vi "Photodetector DAQ (temp).vi"() -> ()   [LabVIEW 2018]
uses:
  <vilib>/DAQmx/read.llb/DAQmx Read (Analog 1D Wfm NChan NSamp).vi
  <vilib>/Analysis/8numeric.llb/1D Numeric Integration.vi
  <vilib>/DAQmx/create/channels.llb/DAQmx Create Channel (AI-Voltage-Basic).vi
  <vilib>/DAQmx/configure/timing.llb/DAQmx Timing (Sample Clock).vi
  <vilib>/DAQmx/configure/trigger.llb/DAQmx Start Trigger (Digital Edge).vi
  <vilib>/DAQmx/miscellaneous.llb/DAQmx Fill In Error Info.vi
  <vilib>/Waveform/WDTOps.llb/WDT Index Channel by Name DBL.vi
  <vilib>/Analysis/NI_AALPro.lvlib
panel:
  out "Minimum of absorption signal":dbl[](graph)
  out "Integral of PMT signal":dbl[](graph)
  out "Waveform Graph":waveform(dbl)[](graph)
  in  "Save data?":bool
  in  "file path (dialog if empty)":path=path "C:/Users/Oskari/Google Drive/CeNTREX Oskari/TlF beam profiling/Data acquisition software/LabView/test.csv"
  out "Error message message":string=" INSTRUCTIONS:\r\rNormal Use:  When using subVIs that incorporate the error in/error out (or error I/O) structure, place this handler where you want to inform the user of an error, typically at the end of the I/O data path, as the last action of the program.  If the error in error? is ERROR, the handler creates a message describing the error and its source.  If the type of dialog = 1 (default), the message is displayed to the user, who can only acknowedge it.  If the type = 2, the user can acknowledge the message or abort execution; aborting a program with active I/O is not recommended.  If the type = 0, no message is displayed; this is used to process the error programmatically, and the error out cluster elements are wired to individual terminals for that reason.  \r\rOther Use:\n\r\nlocal testing.  To test the error code of a subVI or function that does not have the error I/O structure, you can wire its error code and a source string to the local error code and error source inputs.  If error in error? indicates no error and error code is not equal to 0, the local code and source are substituted for the error in values, and error? is set TRUE (ERROR)."
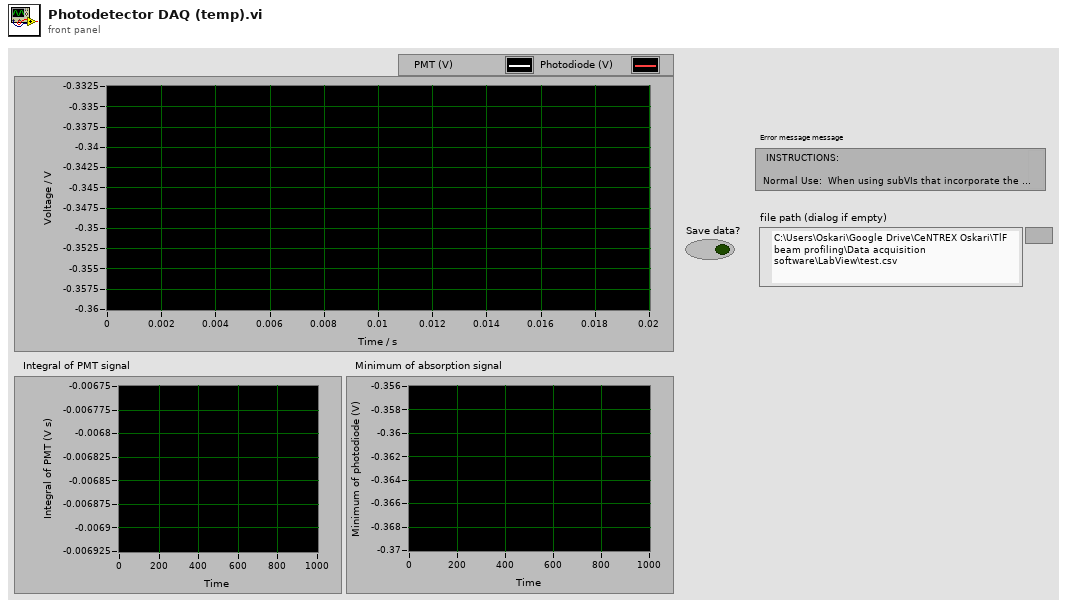
[diagram p1: front panel]
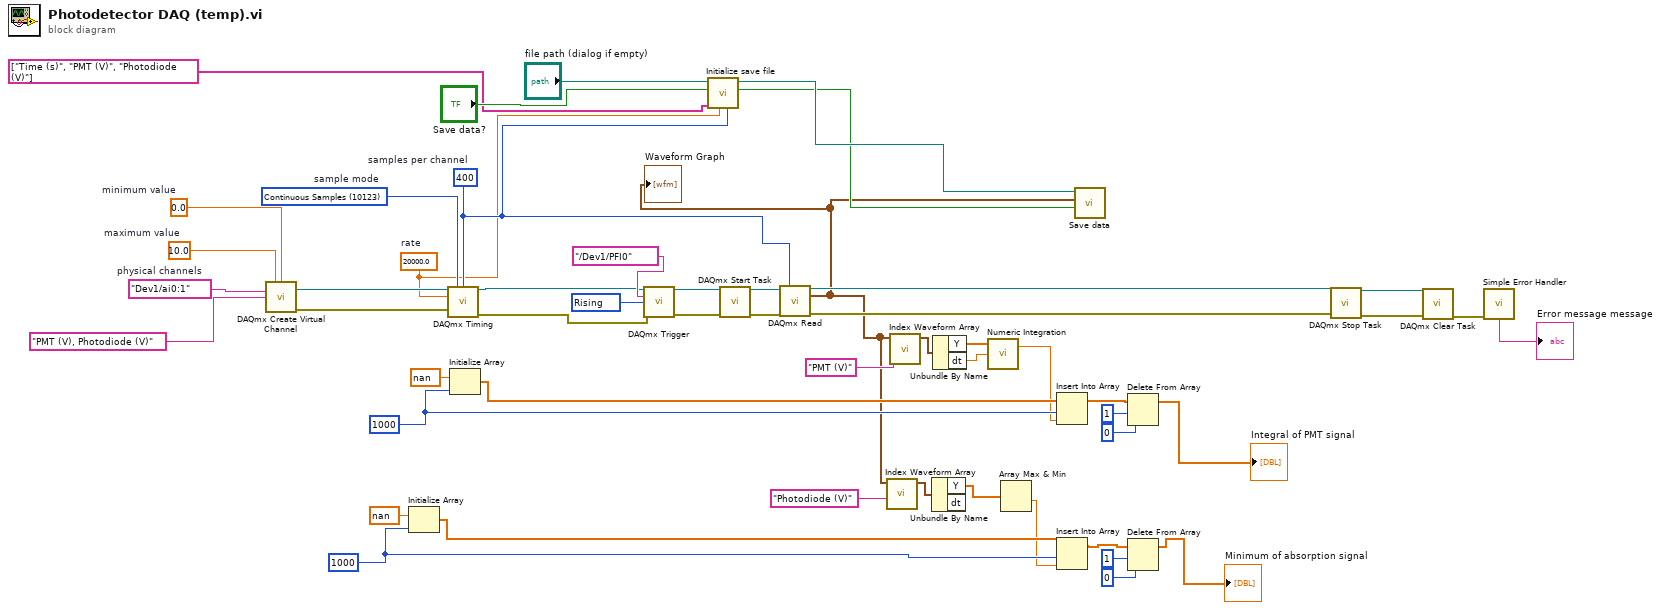
[diagram p0: block diagram]
diagram:
  w27 = 10280 items=["Rising"=10280, "Falling"=10171] ("edge")
  w36 = 1000 ("dimension size")
  w39 = 1000 ("dimension size")
  w31 = 400  # samples per channel
  w47 = 10123 items=["Finite Samples"=10178, "Continuous Samples"=10123, "Hardware Timed Single Point"=12522]  # sample mode
  w30 = 20000.0  # rate
  w50 = 0.0  # minimum value
  w51 = 10.0  # maximum value
  w52 = tag "Dev1/ai0:1"  # physical channels
  n1 = call-poly <vilib>:"DAQmx Create Virtual Channel.vi"("maximum value"=w51, "minimum value"=w50, "physical channels"=w52, "name to assign"="PMT (V), Photodiode (V)") -> ("task out"=w49:refnum<k21>, "error out"=w48:errorcluster)  [unwired: 10 in]
  n2 = Initialize Array(nan ("element"), w36) -> (w37:dbl[])
  n3 = call-poly <vilib>:"DAQmx Timing.vi"("task/channels in"=w49, "sample mode"=w47, "samples per channel"=w31, "rate"=w30, "error in"=w48) -> ("task out"=w6:refnum<k21>, "error out"=w5:errorcluster)  [unwired: 9 in]
  n4 = Initialize Array(nan ("element"), w39) -> (w40:dbl[])
  n5 = call-poly <vilib>:"DAQmx Trigger.vi"("task/channels in"=w6, "source"=tag "/Dev1/PFI0", "edge"=w27, "error in"=w5) -> ("task out"=w3:refnum<k21>, "error out"=w4:errorcluster)  [unwired: 10 in]
  n6 = call "Initialize save file.vi"("Number of samples per channel"=w31, "Sampling rate"=w30, "Headers"=string[] ["Time (s)", "PMT (V)", "Photodiode (V)"], "Save data? in"="Save data?", "Save data path in"="file path (dialog if empty)") -> ("Save data? out"=w33:bool, "Save data path out"=w34:path)  [unwired: 5 in]
  n7 = call <vilib>:"DAQmx Start Task.vi"("task/channels in"=w3, "error in"=w4) -> ("task out"=w2:refnum<k21>, "error out"=w1:errorcluster)  [unwired: 12 in]
  n8 = call-poly <vilib>:"DAQmx Read.vi"("task/channels in"=w2, "number of samples per channel"=w31, "error in"=w1) -> ("task out"=w26:refnum<k21>, "data"=w16:waveform(dbl)[], "error out"=w25:errorcluster)  [unwired: 10 in]
  "Waveform Graph" <- w16
  n9 = call-poly <vilib>:"Index Waveform Array.vi"("channel name"="Photodiode (V)" ("index"), "waveform array"=w16) -> ("waveform"=w14:waveform(dbl))  [unwired: 8 in, 1 out]
  n10 = call-poly <vilib>:"Index Waveform Array.vi"("channel name"="PMT (V)" ("index"), "waveform array"=w16) -> ("waveform"=w23:waveform(dbl))  [unwired: 8 in, 1 out]
  n11 = Unbundle By Name(w14) -> ("Y"=w13:dbl[])  [unwired: 1 out]
  n12 = Unbundle By Name(w23) -> ("Y"=w22:dbl[], "dt"=w21:dbl)
  n13 = call-poly <vilib>:"Numeric Integration.vi"("dt"=w21, "Input Array"=w22) -> ("result"=w20:dbl)  [unwired: 1 in, 1 out]
  n14 = Array Max & Min(array=w13) -> (min value=w12:dbl)  [unwired: 3 out]
  n15 = Insert Into Array(array=w40, index=w39, new element=w20) -> (w19:dbl[])
  n16 = Insert Into Array(array=w37, index=w36, new element=w12) -> (w9:dbl[])
  n17 = call "Save data.vi"("Save data?"=w33, "data"=w16, "file path (dialog if empty)"=w34) -> ()  [unwired: 9 in]
  n18 = Delete From Array(array=w19, length=1, index=0) -> (array with subset deleted=→"Integral of PMT signal":dbl[])  [unwired: 1 out]
  n19 = Delete From Array(array=w9, length=1, index=0) -> (array with subset deleted=→"Minimum of absorption signal":dbl[])  [unwired: 1 out]
  n20 = call <vilib>:"DAQmx Stop Task.vi"("task/channels in"=w26, "error in"=w25) -> ("task out"=w46:refnum<k21>, "error out"=w45:errorcluster)  [unwired: 12 in]
  n21 = call <vilib>:"DAQmx Clear Task.vi"("task in"=w46, "error in"=w45) -> ("error out"=w44:errorcluster)  [unwired: 13 in]
  n22 = call <vilib>:"Simple Error Handler.vi"("error in (no error)"=w44) -> ("message"=→"Error message message":string)  [unwired: 4 in, 4 out]
